vi "Subvi DO mod.vi"(2 "DO channel":refnum<k21>="Connector1/DIO0", 10 "Memory label":refnum<k21>="DO0 buffer") -> ()   [LabVIEW 2017]
uses:
  GV DO delay.vi
  <vilib>/rvi/DataTransferAndStorage/Container/Common/niFpgaContainerExecOnDevCompGetState.vi
  <vilib>/rvi/Emulation/niFpgaEmulationIsFPGAContextNoSignature.vi
  <vilib>/rvi/DataTransferAndStorage/Container/Common/niFpgaContainerGetUniqueNameForEmu.vi
  <vilib>/rvi/Emulation/niFpgaProcessEmulError.vi
  <vilib>/rvi/Emulation/niFpgaSctlEmulationGetInTimedLoop.vi
  <vilib>/rvi/errors/nirviReportUnexpectedCaseInternalError (U32).vi
  <vilib>/rvi/Memory/Memory_Emulation/niFpgaMemoryEmulationCacheClearOnFirstRun.vi
  <vilib>/rvi/Memory/Memory_Emulation/nirvimemoryEmulationManagerCache_MakeExclusive.vi
  <vilib>/rvi/Memory/Memory_Emulation/niFpgaMemoryEmulationValidateCache.vi
  <vilib>/rvi/Memory/Memory_Emulation/nirvimemoryEmulationManagerCache_InsertValue.vi
  <vilib>/Utility/error.llb/Clear Errors.vi
  <vilib>/rvi/Memory/Memory_Emulation/nirvimemoryEmulationManagerCache_ReleaseExclusive.vi
  <vilib>/rvi/Memory/Memory_Emulation/nirvimemoryEmulationManagerCache_GetValue.vi
  <vilib>/rvi/Memory/Memory_Emulation/nirvimemoryEmulationManagerCache_SetValue.vi
  <vilib>/rvi/Emulation/niFpgaSctlEmulationResourceMgr.vi
  <vilib>/rvi/eio/common/nirviEmuTemplateMethod_errors.vi
  <vilib>/rvi/DataTransferAndStorage/Container/XNode/niFpgaContainer.xnode
  <vilib>/rvi/Memory/Memory_Emulation/niFpgaMemoryEmulationRefIn.vi
  <vilib>/eio/EIONode/EIONode.xnode
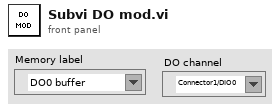
[diagram p1: front panel]
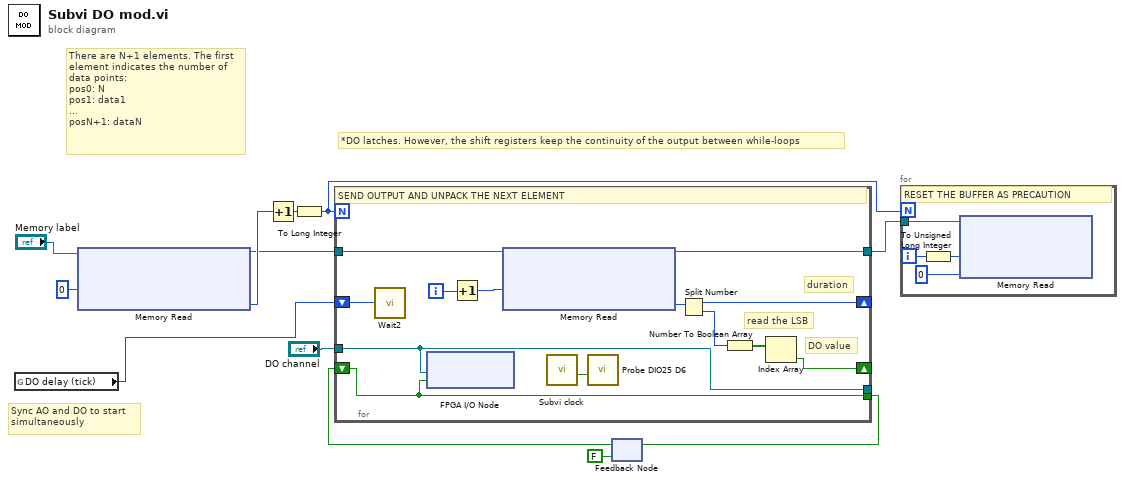
[diagram p0: block diagram]
diagram:
  # "There are N+1 elements. The first\nelement indicates the number of\ndata points:\npos0: N\npos1: data1\n...\nposN+1: dataN"
  # "*DO latches. However, the shift registers keep the continuity of the output between while-loops"
  # "Sync AO and DO to start\nsimultaneously"
  n1 = global read "GV DO delay.vi" "DO delay (tick)"() -> (w2:u16)
  n2 = xnode ("Memory Read")("Memory In"="Memory label", "Address"=u32 0) -> ("Memory Out"=w8:refnum<k21>, "Data"=w10:u32)
  n3 = Increment(x=w10) -> (x+1=w9:u32)
  n4 = To Long Integer(number=w9) -> (32bit integer=w7:i32)
  n5 = feedback #1(FALSE) -> (w5:bool)
  n6 = for {
    N: w7 -> [_]
    shift-right: [w20] -> _
    shift-left: w5 -> [w15]
    shift-right: [w22] -> _
    shift-left: w2 -> [w21]
    tunnel: [w19] -> w11
    tunnel: w8 -> [w18]
    tunnel: [w15] -> w3
    tunnel: "DO channel" -> [w14]
    tunnel: [w14] -> _
    i -> [w17]
    # "read the LSB"
    # "DO value"
    # "duration"
    # "SEND OUTPUT AND UNPACK THE NEXT ELEMENT"
    n7 = call "Wait2"("Count(Ticks)"=w21) -> ()  [unwired: 1 out]
    n8 = xnode "FPGA I/O Node"("I/O Item"=w15, "FPGA I/O In"=w14) -> ()  [unwired: 1 out]
    n9 = Increment(x=w17) -> (x+1=w16:i32)
    n10 = xnode ("Memory Read")("Address"=w16, "Memory In"=w18) -> ("Data"=w24:u32, "Memory Out"=w19:refnum<k21>)
    n11 = call "Subvi clock.vi"() -> ("Output"=w13:bool)  [unwired: 11 in]
    n12 = call "Probe DIO25 D6.vi"("D6"=w13) -> ()  [unwired: 11 in]
    n13 = Split Number(x=w24) -> (hi(x)=w22:u16, lo(x)=w23:u16)
    n14 = Number To Boolean Array(number=w23) -> (Boolean array=w25:bool[])
    n15 = Index Array(array=w25) -> (element=w20:bool)  [unwired: 1 in]
  }
  n16 = feedback-in #1(w3) -> ()
  n17 = for {
    N: w7 -> [_]
    tunnel: w11 -> [w29]
    i -> [w28]
    # "RESET THE BUFFER AS PRECAUTION"
    n18 = To Unsigned Long Integer(number=w28) -> (unsigned 32bit integer=w26:u32)
    n19 = xnode ("Memory Read")("Address"=w26, "Data"=u32 0, "Memory In"=w29) -> ()  [unwired: 1 out]
  }
